vi "find_position.vi"   [LabVIEW 2019]
uses:
  Global Var.vi
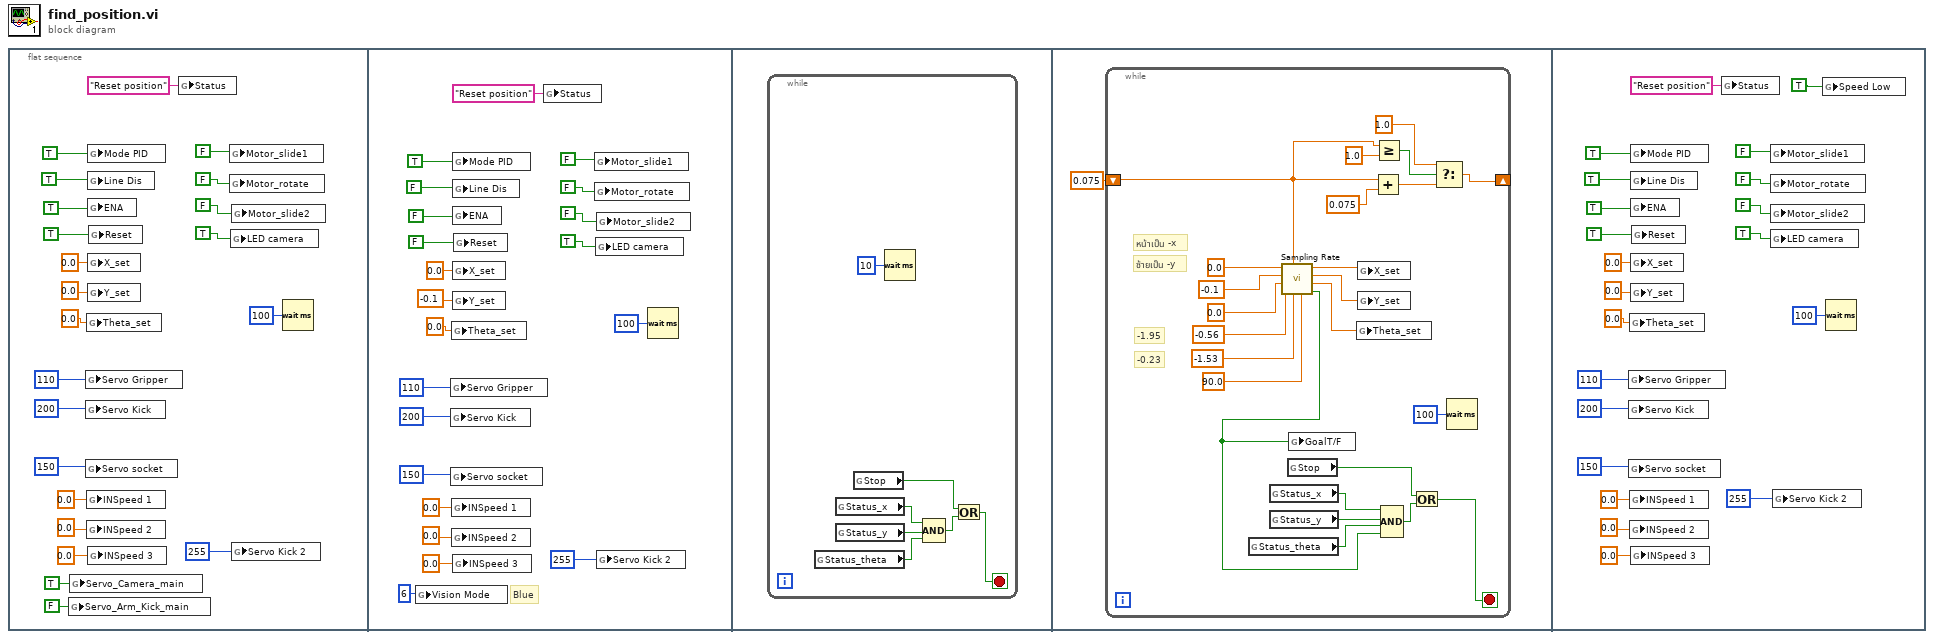
[diagram p0: block diagram]
diagram:
  n1 = flat-sequence {
    frame #0 {
      n2 = global write "Global Var.vi" "Servo_Arm_Kick_main"(FALSE ("Mode PID")) -> ()
      n3 = global write "Global Var.vi" "Servo_Camera_main"(TRUE ("Mode PID")) -> ()
      n4 = global write "Global Var.vi" "Servo Gripper"(u8 110 ("Servo Camera")) -> ()
      n5 = global write "Global Var.vi" "Servo Kick"(u8 200 ("Servo Camera")) -> ()
      n6 = global write "Global Var.vi" "Servo socket"(u8 150 ("Servo Camera")) -> ()
      n7 = global write "Global Var.vi" "Theta_set"(0.0 ("Theta_set")) -> ()
      n8 = global write "Global Var.vi" "INSpeed 1"(0.0 ("X_set")) -> ()
      n9 = global write "Global Var.vi" "INSpeed 2"(0.0 ("Y_set")) -> ()
      n10 = global write "Global Var.vi" "Mode PID"(TRUE ("Mode PID")) -> ()
      n11 = global write "Global Var.vi" "Line Dis"(TRUE ("Mode PID")) -> ()
      n12 = global write "Global Var.vi" "ENA"(TRUE ("ENA")) -> ()
      n13 = global write "Global Var.vi" "X_set"(0.0 ("X_set")) -> ()
      n14 = global write "Global Var.vi" "Y_set"(0.0 ("Y_set")) -> ()
      n15 = global write "Global Var.vi" "INSpeed 3"(0.0 ("Theta_set")) -> ()
      n16 = global write "Global Var.vi" "Reset"(TRUE ("ENA")) -> ()
      n17 = global write "Global Var.vi" "Status"("Reset position" ("Status")) -> ()
      n18 = global write "Global Var.vi" "Motor_slide1"(FALSE ("Mode PID")) -> ()
      n19 = global write "Global Var.vi" "Motor_rotate"(FALSE ("ENA")) -> ()
      n20 = global write "Global Var.vi" "LED camera"(TRUE ("LED camera")) -> ()
      n21 = global write "Global Var.vi" "Motor_slide2"(FALSE ("ENA")) -> ()
      n22 = global write "Global Var.vi" "Servo Kick 2"(u8 255 ("Servo Camera")) -> ()
      n23 = Wait (ms)(milliseconds to wait=u32 100) -> ()  [unwired: 1 out]
    }
    frame #1 {
      # "Blue"
      n24 = global write "Global Var.vi" "Vision Mode"(i16 6 ("Vision Mode")) -> ()
      n25 = global write "Global Var.vi" "Servo Gripper"(u8 110 ("Servo Camera")) -> ()
      n26 = global write "Global Var.vi" "Servo Kick"(u8 200 ("Servo Camera")) -> ()
      n27 = global write "Global Var.vi" "Servo socket"(u8 150 ("Servo Camera")) -> ()
      n28 = global write "Global Var.vi" "Theta_set"(0.0 ("Theta_set")) -> ()
      n29 = global write "Global Var.vi" "INSpeed 1"(0.0 ("X_set")) -> ()
      n30 = global write "Global Var.vi" "INSpeed 2"(0.0 ("Y_set")) -> ()
      n31 = global write "Global Var.vi" "Mode PID"(TRUE ("Mode PID")) -> ()
      n32 = global write "Global Var.vi" "Line Dis"(FALSE ("Mode PID")) -> ()
      n33 = global write "Global Var.vi" "ENA"(FALSE ("ENA")) -> ()
      n34 = global write "Global Var.vi" "X_set"(0.0 ("X_set")) -> ()
      n35 = global write "Global Var.vi" "Y_set"(-0.1 ("Y_set")) -> ()
      n36 = global write "Global Var.vi" "INSpeed 3"(0.0 ("Theta_set")) -> ()
      n37 = global write "Global Var.vi" "Reset"(FALSE ("ENA")) -> ()
      n38 = global write "Global Var.vi" "Status"("Reset position" ("Status")) -> ()
      n39 = global write "Global Var.vi" "Motor_slide1"(FALSE ("Mode PID")) -> ()
      n40 = global write "Global Var.vi" "Motor_rotate"(FALSE ("ENA")) -> ()
      n41 = global write "Global Var.vi" "LED camera"(TRUE ("LED camera")) -> ()
      n42 = global write "Global Var.vi" "Motor_slide2"(FALSE ("ENA")) -> ()
      n43 = global write "Global Var.vi" "Servo Kick 2"(u8 255 ("Servo Camera")) -> ()
      n44 = Wait (ms)(milliseconds to wait=u32 100) -> ()  [unwired: 1 out]
    }
    frame #2 {
      n45 = while {
        stop <- w46 stop-if-true
        n46 = global read "Global Var.vi" "Status_theta"() -> (w48:bool)
        n47 = global read "Global Var.vi" "Status_x"() -> (w49:bool)
        n48 = global read "Global Var.vi" "Status_y"() -> (w50:bool)
        n49 = global read "Global Var.vi" "Stop"() -> (w44:bool)
        n50 = Wait (ms)(milliseconds to wait=u32 10) -> ()  [unwired: 1 out]
        n51 = Compound Arithmetic op=AND(w49, w50, w48) -> (w45:bool)
        n52 = Or(x=w44, y=w45) -> (x .or. y?=w46:bool)
      }
    }
    frame #3 {
      n53 = while {
        shift-right: [w54] -> _
        shift-left: 0.075 -> [w52]
        stop <- w71 stop-if-true
        # "-0.23"
        # "-1.95"
        # "ซ้ายเป็น -y"
        # "หน้าเป็น -x"
        n54 = global read "Global Var.vi" "Status_theta"() -> (w73:bool)
        n55 = global read "Global Var.vi" "Status_x"() -> (w74:bool)
        n56 = global read "Global Var.vi" "Status_y"() -> (w75:bool)
        n57 = call "Sampling Rate.vi"("input a1"=90.0, "input y1"=-1.53, "T(0-1)"=w52, "input x1"=-0.56, "input a0"=0.0, "input y0"=-0.1, "input x0"=0.0) -> ("GoalT/F"=w59:bool, "a_output"=w66:dbl, "y_output"=w67:dbl, "x_output"=w68:dbl)  [unwired: 1 in]
        n58 = global read "Global Var.vi" "Stop"() -> (w69:bool)
        n59 = global write "Global Var.vi" "GoalT/F"(w59) -> ()
        n60 = global write "Global Var.vi" "Theta_set"(w66) -> ()
        n61 = global write "Global Var.vi" "X_set"(w68) -> ()
        n62 = global write "Global Var.vi" "Y_set"(w67) -> ()
        n63 = Add(x=w52, y=0.075) -> (x+y=w57:dbl)
        n64 = Greater Or Equal?(x=w52, y=1.0) -> (x >= y?=w56:bool)
        n65 = Compound Arithmetic op=AND(w74, w75, w73, w59) -> (w70:bool)
        n66 = Or(x=w69, y=w70) -> (x .or. y?=w71:bool)
        n67 = Select(t=1.0, s=w56, f=w57) -> (s? t:f=w54:dbl)
        n68 = Wait (ms)(milliseconds to wait=u32 100) -> ()  [unwired: 1 out]
      }
    }
    frame #4 {
      n69 = global write "Global Var.vi" "Servo Gripper"(u8 110 ("Servo Camera")) -> ()
      n70 = global write "Global Var.vi" "Servo Kick"(u8 200 ("Servo Camera")) -> ()
      n71 = global write "Global Var.vi" "Servo socket"(u8 150 ("Servo Camera")) -> ()
      n72 = global write "Global Var.vi" "Theta_set"(0.0 ("Theta_set")) -> ()
      n73 = global write "Global Var.vi" "INSpeed 1"(0.0 ("X_set")) -> ()
      n74 = global write "Global Var.vi" "INSpeed 2"(0.0 ("Y_set")) -> ()
      n75 = global write "Global Var.vi" "Mode PID"(TRUE ("Mode PID")) -> ()
      n76 = global write "Global Var.vi" "Line Dis"(TRUE ("Mode PID")) -> ()
      n77 = global write "Global Var.vi" "ENA"(TRUE ("ENA")) -> ()
      n78 = global write "Global Var.vi" "X_set"(0.0 ("X_set")) -> ()
      n79 = global write "Global Var.vi" "Y_set"(0.0 ("Y_set")) -> ()
      n80 = global write "Global Var.vi" "INSpeed 3"(0.0 ("Theta_set")) -> ()
      n81 = global write "Global Var.vi" "Reset"(TRUE ("ENA")) -> ()
      n82 = global write "Global Var.vi" "Status"("Reset position" ("Status")) -> ()
      n83 = global write "Global Var.vi" "Motor_slide1"(FALSE ("Mode PID")) -> ()
      n84 = global write "Global Var.vi" "Motor_rotate"(FALSE ("ENA")) -> ()
      n85 = global write "Global Var.vi" "Motor_slide2"(FALSE ("ENA")) -> ()
      n86 = global write "Global Var.vi" "LED camera"(TRUE ("LED camera")) -> ()
      n87 = global write "Global Var.vi" "Servo Kick 2"(u8 255 ("Servo Camera")) -> ()
      n88 = global write "Global Var.vi" "Speed Low"(TRUE ("LED camera")) -> ()
      n89 = Wait (ms)(milliseconds to wait=u32 100) -> ()  [unwired: 1 out]
    }
  }
